vi "Generate Simulated Data.vi"(6 "Acquisition":refnum<queue>, 8 "error in (no error)":errorcluster, 10 "Longueur d'onde":dbl) -> (0 "error out":errorcluster, 2 "Data Out":variant[](array[variant]), 3 "Disconnected":bool=TRUE)   [LabVIEW 2018, in "Acquisition.lvlib"]
doc: "Generates sample waveforms according to the signal type in the HW Config input."
uses:
  Acquisition.lvlib
  <vilib>/Analysis/NI_AALBase.lvlib
  GlobalVariable/GlobalPowerByTime.vi
  GlobalVariable/Globalt0.vi
  support/Message Queue/Message Queue.lvlib
  <vilib>/gmath/NI_Gmath.lvlib
  GlobalVariable/GlobalSet0.vi
  <vilib>/Analysis/NI_AALPro.lvlib
  GlobalVariable/GlobalPosXbyTime.vi
  GlobalVariable/GlobalPosYbyTime.vi
  GlobalVariable/GlobalProfileByTime.vi
  GlobalVariable/GlobalTimeStep.vi
  GlobalVariable/GlobalTensionByTime.vi
  GlobalVariable/GlobalTemperatureByTime.vi
  support/Message Queue/Enqueue Message (Single).vi
  <vilib>/gmath/interp.llb/Create Mesh Grid (2D) (x,y arrays).vi
  <vilib>/Analysis/2dsp.llb/2D Convolution (DBL).vi
  <vilib>/Analysis/baseanly.llb/Mean (DBL).vi
  <vilib>/DAQmx/create/channels.llb/DAQmx Create Channel (DO-Digital Output).vi
  <resource>/objmgr/daqmx.rc
  <vilib>/DAQmx/write.llb/DAQmx Write (Digital 1D Bool NChan 1Samp 1Line).vi
  <vilib>/DAQmx/create/channels.llb/DAQmx Create Channel (AI-Voltage-Basic).vi
  <vilib>/DAQmx/configure/timing.llb/DAQmx Timing (Sample Clock).vi
  <vilib>/DAQmx/read.llb/DAQmx Read (Analog 1D Wfm NChan NSamp).vi
  support/Message Queue/Message Cluster.ctl
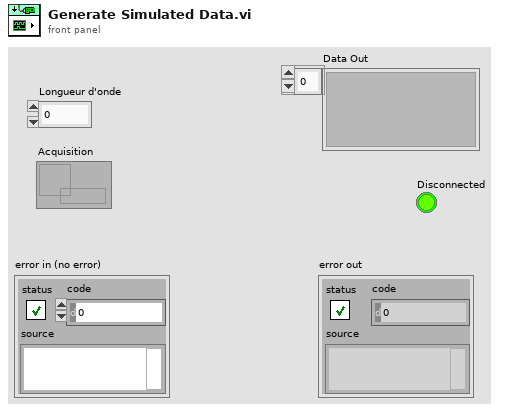
[diagram p1: front panel]
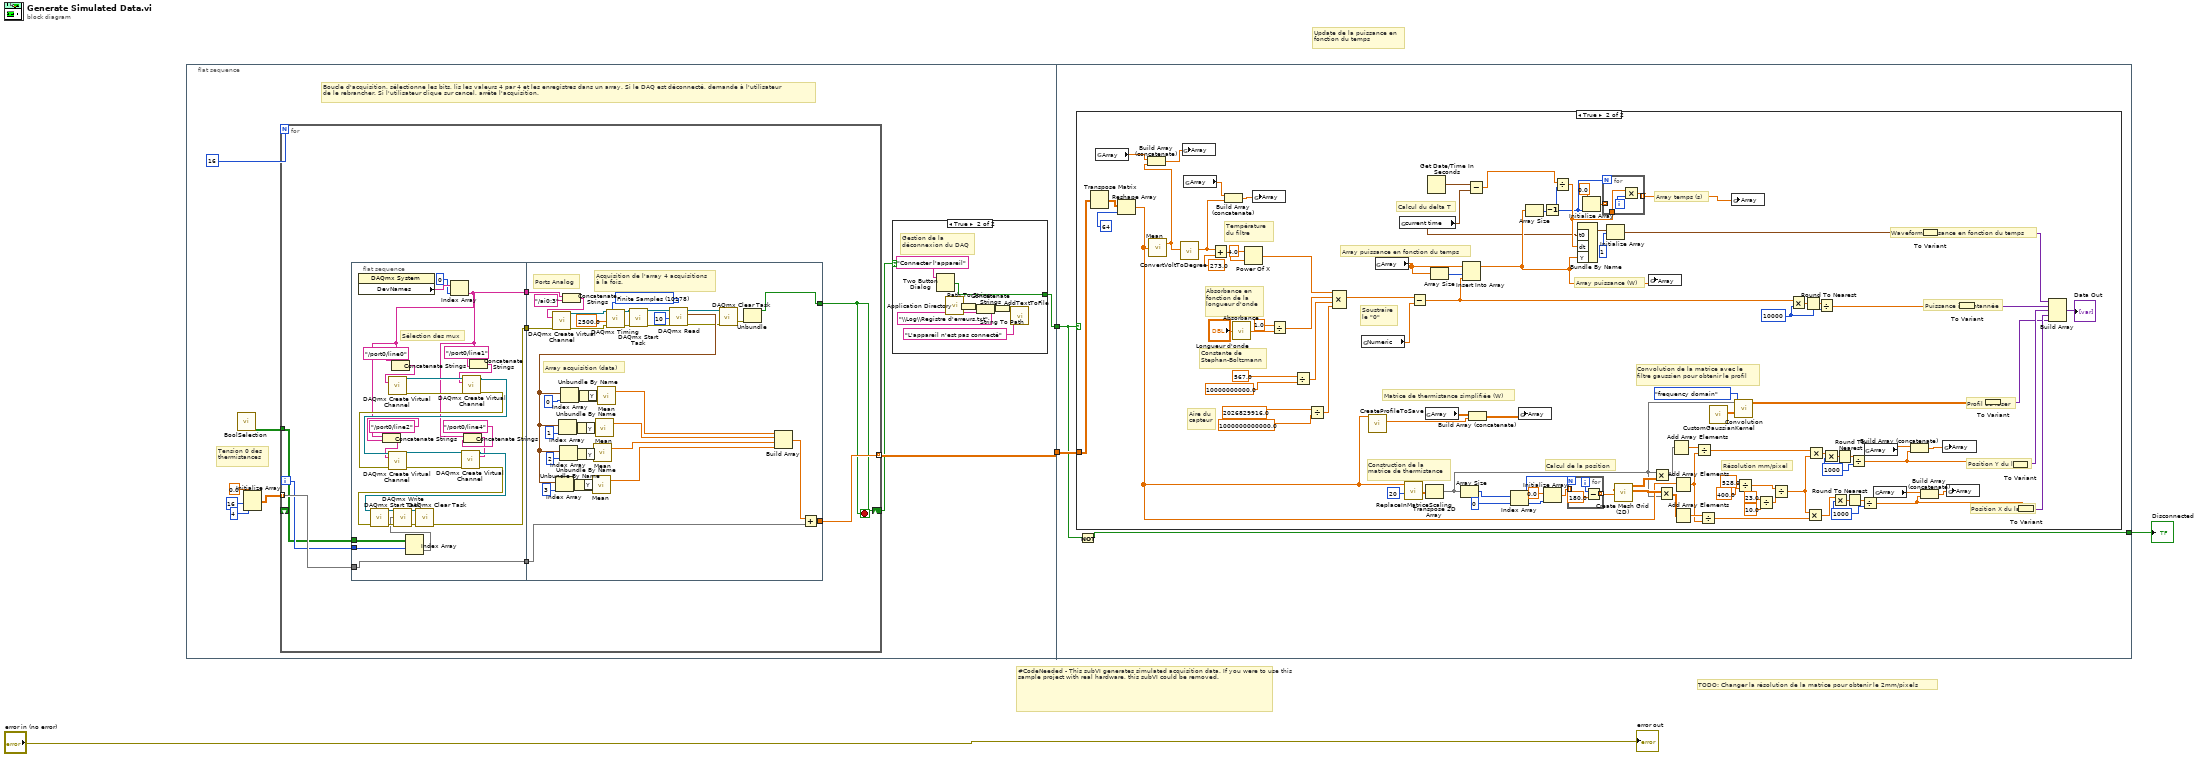
[diagram p0: block diagram]
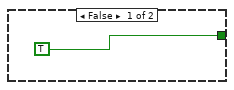
[diagram p2: hidden frame]
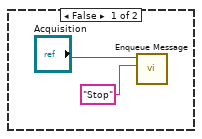
[diagram p3: hidden frame]
diagram:
  # "TODO: Changer la résolution de la matrice pour obtenir le 2mm/pixels"
  # "Update de la puissance en\nfonction du temps"
  # "#CodeNeeded - This subVI generates simulated acquisition data. If you were to use this sample project with real hardware, this subVI could be removed."
  n1 = flat-sequence {
    tunnel: [w11] -> w3
    tunnel: [w10] -> w2
    tunnel: w3 -> [w98]
    tunnel: w2 -> [w97]
    tunnel: [w96] -> w1
    frame #0 {
      # "Boucle d'acquisition, sélectionne les bits, lis les valeurs 4 par 4 et les enregistres dans un array. Si le DAQ est déconnecté, demande à l'utilisateur \nde le rebrancher. Si l'utilisateur clique sur cancel, arrête l'acquisition."
      # "Tension 0 des \nthermistances"
      n2 = call "BoolSelection.vi"() -> ("BoolSelection"=w12:bool[][])  [unwired: 11 in]
      n3 = Initialize Array(0.0 ("element"), 16 ("dimension size"), 4 ("dimension size")) -> (w6:dbl[][])
      n4 = for {
        N: 16 -> [_]
        tunnel: w12 -> [w25]
        tunnel: w6 -> [w30] mode=indexing
        tunnel: [w24] -> w11 mode=indexing
        shift-right: [w23] -> w5
        shift-left: _ -> [_]
        i -> [w26]
        stop <- w23 stop-if-true
        n5 = flat-sequence {
          tunnel: w26 -> [w44]
          tunnel: [w55] -> w29
          tunnel: w25 -> [w43]
          tunnel: [w31] -> w28
          tunnel: [w32] -> w27
          tunnel: w30 -> [w31]
          tunnel: w29 -> [w87]
          tunnel: w28 -> [w67]
          tunnel: [w69] -> w24
          tunnel: w27 -> [w64]
          tunnel: [w59] -> w23
          frame #0 {
            # "Sélection des mux"
            n6 = property class="DAQmx System"() -> ("DevNames"=w42:tag[])  [unwired: 2 in, 2 out]
            n7 = Index Array(array=w43, index (row)=w44) -> (element=w56:bool[])  [unwired: 1 in]
            n8 = Index Array(array=w42, index=0) -> (element=w32:tag)
            n9 = Concatenate Strings(w32, "/port0/line2" ("string")) -> (w35:string)
            n10 = Concatenate Strings(w32, "/port0/line0" ("string")) -> (w40:string)
            n11 = call-poly <vilib>:"DAQmx Create Virtual Channel.vi"("lines"=w40) -> ("task out"=w51:refnum<k21>, "error out"=w52:errorcluster)  [unwired: 13 in]
            n12 = Concatenate Strings(w32, "/port0/line4" ("string")) -> (w33:string)
            n13 = Concatenate Strings(w32, "/port0/line1" ("string")) -> (w37:string)
            n14 = call-poly <vilib>:"DAQmx Create Virtual Channel.vi"("task in"=w51, "lines"=w37, "error in"=w52) -> ("task out"=w50:refnum<k21>, "error out"=w49:errorcluster)  [unwired: 11 in]
            n15 = call-poly <vilib>:"DAQmx Create Virtual Channel.vi"("task in"=w50, "lines"=w35, "error in"=w49) -> ("task out"=w47:refnum<k21>, "error out"=w48:errorcluster)  [unwired: 11 in]
            n16 = call-poly <vilib>:"DAQmx Create Virtual Channel.vi"("task in"=w47, "lines"=w33, "error in"=w48) -> ("task out"=w46:refnum<k21>, "error out"=w45:errorcluster)  [unwired: 11 in]
            n17 = call <vilib>:"DAQmx Start Task.vi"("task/channels in"=w46, "error in"=w45) -> ("task out"=w57:refnum<k21>, "error out"=w58:errorcluster)  [unwired: 12 in]
            n18 = call-poly <vilib>:"DAQmx Write.vi"("task/channels in"=w57, "data"=w56, "error in"=w58) -> ("task out"=w54:refnum<k21>, "error out"=w53:errorcluster)  [unwired: 10 in, 1 out]
            n19 = call <vilib>:"DAQmx Clear Task.vi"("task in"=w54, "error in"=w53) -> ("error out"=w55:errorcluster)  [unwired: 13 in]
          }
          frame #1 {
            w89 = 10178 items=["Finite Samples"=10178, "Continuous Samples"=10123, "Hardware Timed Single Point"=12522] ("sample mode")
            # "Ports Analog"
            # "Array acquisition (data)"
            # "Acquisition de l'array 4 acquisitions\nà la fois."
            n20 = Concatenate Strings(w64, "/ai0:3" ("string")) -> (w65:string)
            n21 = call-poly <vilib>:"DAQmx Create Virtual Channel.vi"("physical channels"=w65, "error in"=w87) -> ("task out"=w94:refnum<k21>, "error out"=w93:errorcluster)  [unwired: 12 in]
            n22 = call-poly <vilib>:"DAQmx Timing.vi"("task/channels in"=w94, "sample mode"=w89, "rate"=2500.0, "error in"=w93) -> ("task out"=w90:refnum<k21>, "error out"=w91:errorcluster)  [unwired: 10 in]
            n23 = call <vilib>:"DAQmx Start Task.vi"("task/channels in"=w90, "error in"=w91) -> ("task out"=w92:refnum<k21>, "error out"=w95:errorcluster)  [unwired: 12 in]
            n24 = call-poly <vilib>:"DAQmx Read.vi"("task/channels in"=w92, "number of samples per channel"=10, "error in"=w95) -> ("task out"=w71:refnum<k21>, "data"=w80:waveform(dbl)[], "error out"=w70:errorcluster)  [unwired: 10 in]
            n25 = Index Array(array=w80, index=3) -> (element=w76:waveform(dbl))
            n26 = Index Array(array=w80, index=1) -> (element=w78:waveform(dbl))
            n27 = Index Array(array=w80, index=2) -> (element=w77:waveform(dbl))
            n28 = Index Array(array=w80, index=0) -> (element=w79:waveform(dbl))
            n29 = Unbundle By Name(w76) -> ("Y"=w72:dbl[])
            n30 = Unbundle By Name(w78) -> ("Y"=w74:dbl[])
            n31 = Unbundle By Name(w77) -> ("Y"=w73:dbl[])
            n32 = Unbundle By Name(w79) -> ("Y"=w75:dbl[])
            n33 = call-poly <vilib>:"Mean.vi"("X"=w72) -> ("mean"=w60:dbl)  [unwired: 1 out]
            n34 = call-poly <vilib>:"Mean.vi"("X"=w73) -> ("mean"=w61:dbl)  [unwired: 1 out]
            n35 = call-poly <vilib>:"Mean.vi"("X"=w74) -> ("mean"=w62:dbl)  [unwired: 1 out]
            n36 = call-poly <vilib>:"Mean.vi"("X"=w75) -> ("mean"=w63:dbl)  [unwired: 1 out]
            n37 = call <vilib>:"DAQmx Clear Task.vi"("task in"=w71, "error in"=w70) -> ("error out"=w85:errorcluster)  [unwired: 13 in]
            n38 = Unbundle(w85) -> ("status"=w59:bool)  [unwired: 2 out]
            n39 = Build Array(w63, w62, w61, w60) -> (w68:dbl[])
            n40 = Add(x=w68, y=w67) -> (x+y=w69:dbl[])
          }
        }
      }
      n41 = case shown="True" w5 {
        tunnel: [TRUE w22] -> w10
        frame False {
        }
        frame True {
          # "Gestion de la \ndéconnexion du DAQ"
          n42 = Two Button Dialog(message="Connecter l'appareil") -> (T button?=w22:bool)  [unwired: 2 in]
          n43 = call <vilib>:"Application Directory.vi"() -> ("Application Directory"=w19:path)
          n44 = Path To String(path=w19) -> (string=w20:string)
          n45 = Concatenate Strings(w20, "\\Log\\Registre d'erreurs.txt") -> (w21:string)
          n46 = String To Path(string=w21) -> (path=w17:path)
          n47 = call "AddTextToFile.vi"("Ajouter du texte"="L'appareil n'est pas connecté", "Fichier"=w17) -> ()  [unwired: 10 in]
        }
      }
    }
    frame #1 {
      n48 = case shown="True" w97 {
        tunnel: w98 -> [_ w137]
        frame False {
          n49 = call-poly "Enqueue Message.vi"("Message"="Stop", "Message Queue"="Acquisition") -> ()  [unwired: 8 in, 2 out]
        }
        frame True {
          w147 = 1000
          w151 = 1000
          w157 = 10000
          # "Résolution mm/pixel"
          # "Calcul du delta T"
          # "Matrice de thermistance simplifiée (W)"
          # "Soustraire\nle \"0\""
          # "Constante de \nStephan-Boltzmann"
          # "Absorbance en\nfonction de la \nlongueur d'onde"
          # "Température \ndu filtre"
          # "Aire du\ncapteur"
          # "Calcul de la position"
          # "Construction de la \nmatrice de thermistance"
          # "Position X du laser"
          # "Position Y du laser"
          # "Profil du laser"
          # "Puissance instantannée"
          # "Waveform puissance en fonction du temps"
          # "Array puissance (W)"
          # "Array temps (s)"
          # "Convolution de la matrice avec le \nfiltre gaussien pour obtenir le profil"
          # "Array puissance en fonction du temps"
          n50 = Transpose Matrix(1:w137) -> (0:w138:dbl[][])
          n51 = global read "GlobalTensionByTime.vi" "Array"() -> (w116:dbl[])
          n52 = Reshape Array(w138, 64 ("dimension size")) -> (w133:dbl[])
          n53 = call-poly <vilib>:"Mean.vi"("X"=w133) -> ("mean"=w114:dbl)  [unwired: 1 out]
          n54 = Build Array (concatenate)(w116, w114) -> (w115:dbl[])
          n55 = call "ConvertVoltToDegree.vi"("Tension"=w114) -> ("Température"=w111:dbl)  [unwired: 10 in]
          n56 = global write "GlobalTensionByTime.vi" "Array"(w115) -> ()
          n57 = global read "GlobalTemperatureByTime.vi" "Array"() -> (w112:dbl[])
          n58 = Add(x=w111, y=273.0) -> (x+y=w185:dbl)
          n59 = Build Array (concatenate)(w112, w111) -> (w113:dbl[])
          n60 = call "Absorbance.vi"("Longueur d'onde"="Longueur d'onde") -> ("absorbance"=w102:dbl)  [unwired: 10 in]
          n61 = Power Of X(1:w185, 2:4.0 ("y")) -> (0:w140:dbl)
          n62 = global write "GlobalTemperatureByTime.vi" "Array"(w113) -> ()
          n63 = Divide(x=1.0, y=w102) -> (x/y=w101:dbl)
          n64 = Divide(x=567.0, y=10000000000.0) -> (x/y=w141:dbl)
          n65 = Divide(x=2026829916.0, y=1000000000000.0) -> (x/y=w142:dbl)
          n66 = Compound Arithmetic op=MULTIPLY(w140, w101, w141, w142) -> (w136:dbl)
          n67 = global read "GlobalSet0.vi" "Numeric"() -> (w135:dbl)
          n68 = call "CreateProfileToSave.vi"("Input Array"=w133) -> ("Ouput array"=w123:dbl[])  [unwired: 10 in]
          n69 = global read "GlobalPowerByTime.vi" "Array"() -> (w197:dbl[])
          n70 = global read "Globalt0.vi" "current time"() -> (w118:timestamp)
          n71 = call "ReplaceInMatriceScaling.vi"("Input Scaling"=20, "Input Array"=w133) -> ("Output Array"=w192:dbl[][])  [unwired: 9 in]
          n72 = Subtract(x=w136, y=w135) -> (x-y=w134:dbl)
          n73 = global read "GlobalProfileByTime.vi" "Array"() -> (w122:dbl[][])
          n74 = Transpose 2D Array(2D array=w192) -> (transposed array=w105:dbl[][])
          n75 = Get Date/Time In Seconds() -> (seconds since 1Jan1904=w119:timestamp)
          n76 = Array Size(array=w197) -> (size(s)=w196:i32)
          n77 = Array Size(array=w105) -> (size(s)=w179:i32[])
          n78 = Insert Into Array(array=w197, index=w196, new element=w134) -> (w132:dbl[])
          n79 = Subtract(x=w119, y=w118) -> (x-y=w117:dbl)
          n80 = Build Array (concatenate)(w122, w123) -> (w124:dbl[][])
          n81 = Index Array(array=w179, index=0) -> (element=w174:i32)
          n82 = global write "GlobalProfileByTime.vi" "Array"(w124) -> ()
          n83 = Array Size(array=w132) -> (size(s)=w121:i32)
          n84 = Decrement(x=w121) -> (x-1=w120:i32)
          n85 = Initialize Array(0.0 ("element"), w174) -> (w176:dbl[])
          n86 = Divide(x=w117, y=w120) -> (x/y=w190:dbl)
          n87 = for {
            N: w174 -> [_]
            tunnel: w176 -> [_] mode=indexing
            tunnel: [w198] -> w171 mode=indexing
            i -> [w199]
            n88 = Subtract(x=w199, y=180.0) -> (x-y=w198:dbl)
          }
          n89 = Bundle By Name("t0"=w118, "dt"=w190, "Y"=w132) -> (w194:waveform(dbl))  [unwired: 1 in]
          n90 = Initialize Array(0.0 ("element"), w120) -> (w188:dbl[])
          n91 = for {
            N: w120 -> [_]
            tunnel: w190 -> [w202]
            tunnel: w188 -> [_] mode=indexing
            tunnel: [w201] -> w131 mode=indexing
            i -> [w203]
            n92 = Multiply(x=w202, y=w203) -> (x*y=w201:dbl)
          }
          n93 = Initialize Array(w194, 1) -> (w161:waveform(dbl)[])
          n94 = call-poly <vilib>:"Create Mesh Grid (2D).vi"("y domain"=w171, "x domain"=w171) -> ("Y"=w170:dbl[][], "X"=w175:dbl[][])  [unwired: 7 in, 1 out]
          n95 = global write "GlobalPowerByTime.vi" "Array"(w132) -> ()
          n96 = Multiply(x=w105, y=w175) -> (x*y=w173:dbl[][])
          n97 = Multiply(x=w170, y=w105) -> (x*y=w169:dbl[][])
          n98 = Add Array Elements(numeric array=w173) -> (sum=w172:dbl)
          n99 = Add Array Elements(numeric array=w133) -> (sum=w167:dbl)
          n100 = Add Array Elements(numeric array=w169) -> (sum=w168:dbl)
          n101 = Divide(x=w172, y=w167) -> (x/y=w165:dbl)
          n102 = Divide(x=w168, y=w167) -> (x/y=w166:dbl)
          n103 = call "CustomGaussianKernel.vi"() -> ("array"=w187:dbl[][])  [unwired: 11 in]
          n104 = global write "GlobalTimeStep.vi" "Array"(w131) -> ()
          n105 = call-poly <vilib>:"Convolution.vi"("algorithm"=enum32{"direct", "frequency domain"}."frequency domain", "Y"=w187, "X"=w105) -> ("X * Y"=w104:dbl[][])  [unwired: 7 in, 1 out]
          n106 = Divide(x=528.0, y=400.0) -> (x/y=w108:dbl)
          n107 = Divide(x=23.0 ("y"), y=10.0) -> (x/y=w107:dbl)
          n108 = Divide(x=w108, y=w107) -> (x/y=w106:dbl)
          n109 = Multiply(x=w134, y=w157) -> (x*y=w158:dbl)
          n110 = Round To Nearest(number=w158) -> (nearest integer value=w156:dbl)
          n111 = Multiply(x=w106, y=w166) -> (x*y=w144:dbl)
          n112 = Multiply(x=w165, y=w106) -> (x*y=w148:dbl)
          n113 = Divide(x=w156, y=w157) -> (x/y=w152:dbl)
          n114 = Multiply(x=w148, y=w151) -> (x*y=w150:dbl)
          n115 = Multiply(x=w144, y=w147) -> (x*y=w146:dbl)
          n116 = Round To Nearest(number=w150) -> (nearest integer value=w149:dbl)
          n117 = Round To Nearest(number=w146) -> (nearest integer value=w145:dbl)
          n118 = Divide(x=w149, y=w151) -> (x/y=w125:dbl)
          n119 = Divide(x=w145, y=w147) -> (x/y=w129:dbl)
          n120 = global read "GlobalPosXbyTime.vi" "Array"() -> (w126:dbl[])
          n121 = global read "GlobalPosYbyTime.vi" "Array"() -> (w130:dbl[])
          n122 = Build Array (concatenate)(w126, w125) -> (w127:dbl[])
          n123 = Build Array (concatenate)(w130, w129) -> (w128:dbl[])
          n124 = To Variant(anything=w161) -> (Variant=w160:variant)
          n125 = global write "GlobalPosXbyTime.vi" "Array"(w127) -> ()
          n126 = global write "GlobalPosYbyTime.vi" "Array"(w128) -> ()
          n127 = To Variant(anything=w152) -> (Variant=w153:variant)
          n128 = To Variant(anything=w104) -> (Variant=w143:variant)
          n129 = To Variant(anything=w125) -> (Variant=w154:variant)
          n130 = To Variant(anything=w129) -> (Variant=w155:variant)
          n131 = Build Array(w160, w153, w154, w155, w143) -> (→"Data Out":variant[])
        }
      }
      n132 = Not(x=w97) -> (.not. x?=w96:bool)
    }
  }
  "error out" <- "error in (no error)"
  "Disconnected" <- w1
